vi "Current_Calib_Filenames.vi"(3 "Calib Filename":path[](array[path]), 4 "Channel ID input":string[](array[string]), 5 "Mode":T1) -> (0 "Calib Filename Out":path[](array[path]), 1 "Channel ID Output":string[](array[string]))   [LabVIEW 2017]
uses:
  Controls/App_Global.ctl
  File/Setup_Filetype.ctl
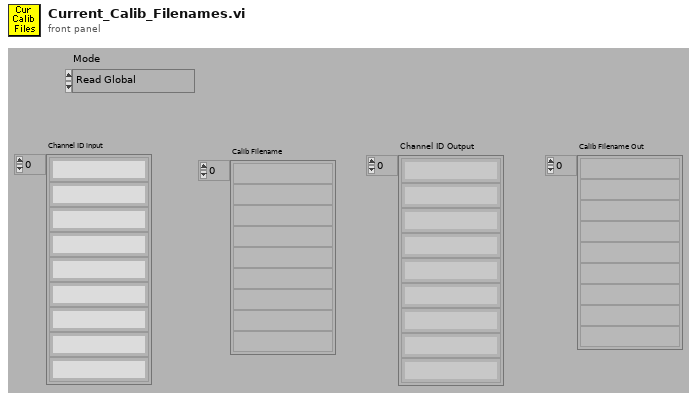
[diagram p1: front panel]
types:
  T1 = typedef "App_Global.ctl" = enum16{"Read Global", "Write to Global", "Initialise Array"}
  T2 = typedef "Setup_Filetype.ctl" = enum16{"Measurement Setups", "Calibration Setups", "General", "Results File Plotter Setups", "Speed Calib Tweaks"}
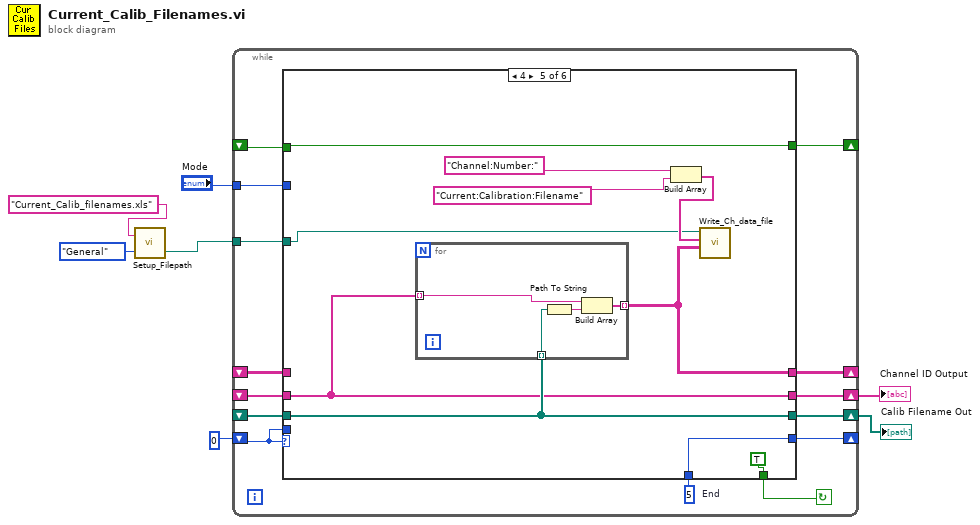
[diagram p0: block diagram]
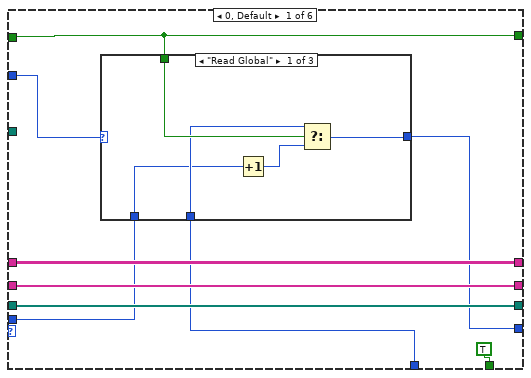
[diagram p2: hidden frame]
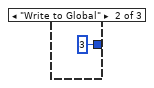
[diagram p3: hidden frame]
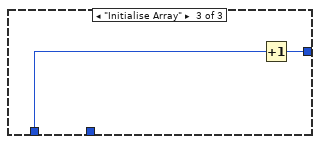
[diagram p4: hidden frame]
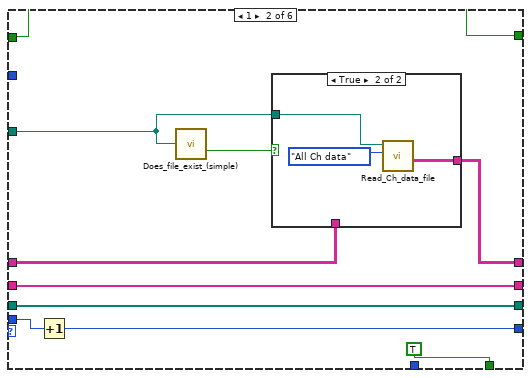
[diagram p5: hidden frame]
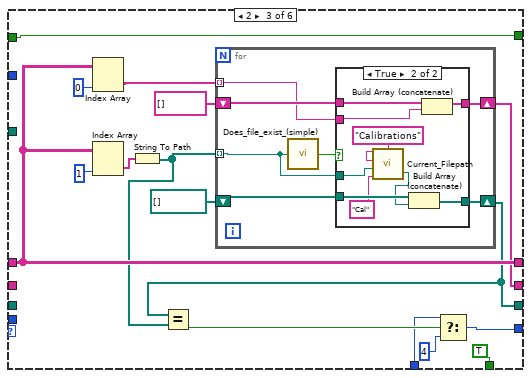
[diagram p7: hidden frame]
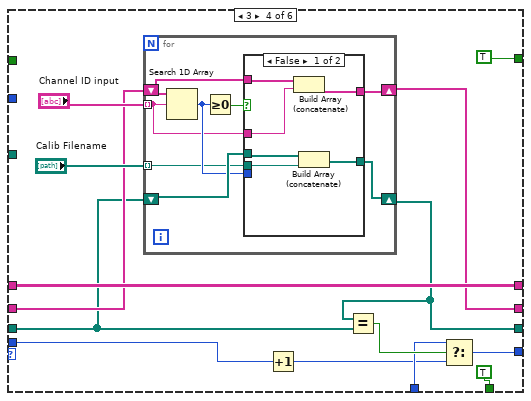
[diagram p9: hidden frame]
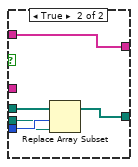
[diagram p10: hidden frame]
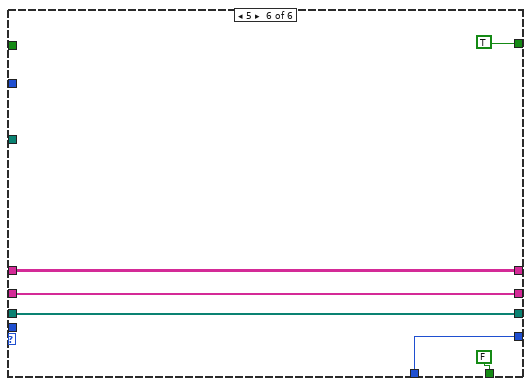
[diagram p11: hidden frame]
diagram:
  n1 = call "Setup_Filepath.vi"("Setup File Type"=Setup_Filetype."General", "Filename in"="Current_Calib_filenames.xls" ("Substring")) -> ("Filename Out"=w2:path)  [unwired: 1 out]
  n2 = while {
    shift-left: _ -> [w10]
    shift-right: [w12] -> w4
    shift-left: _ -> [w11]
    shift-right: [w13] -> w5
    tunnel: "Mode" -> [w17]
    shift-left: 0 -> [w18]
    shift-right: [w19] -> _
    shift-left: _ -> [w14]
    shift-right: [w15] -> _
    shift-left: _ -> [w21]
    shift-right: [w16] -> _
    tunnel: w2 -> [w8]
    stop <- w20 continue-if-true
    w9 = 5  # End
    n3 = case shown="4" w18 {
      tunnel: w21 -> [w25 w45 w64 _ w129 _]
      tunnel: [TRUE TRUE TRUE TRUE TRUE FALSE] -> w20
      tunnel: [w22 w46 w56 w87 w128 w135] -> w19
      tunnel: w18 -> [w23 w47 _ w89 _ _]
      tunnel: w17 -> [w26 _ _ _ _ _]
      tunnel: [w25 w45 w64 TRUE w129 TRUE] -> w16
      tunnel: [w28 w43 w63 w99 w121 w138] -> w15
      tunnel: w14 -> [w28 w42 w63 w99 _ w138]
      tunnel: [w30 w41 w61 w94 w122 w137] -> w13
      tunnel: [w29 w40 w60 w93 w123 w136] -> w12
      tunnel: w11 -> [w30 w41 _ w95 w122 w137]
      tunnel: w10 -> [w29 w40 _ w92 w123 w136]
      tunnel: w9 -> [w24 _ w57 w90 w128 w135]
      tunnel: w8 -> [_ w39 _ _ w120 _]
      frame 0, Default {
        n4 = case shown="\"Read Global\"" w26 {
          tunnel: w25 -> [w35 _ _]
          tunnel: w24 -> [w34 _ _]
          tunnel: w23 -> [w32 _ w38]
          tunnel: [w31 3 ("End") w37] -> w22
          frame "Read Global" {
            n5 = Increment(x=w32) -> (x+1=w33:i32)
            n6 = Select(t=w34, s=w35, f=w33) -> (s? t:f=w31:i32)
          }
          frame "Write to Global" {
          }
          frame "Initialise Array" {
            n7 = Increment(x=w38) -> (x+1=w37:i32)
          }
        }
      }
      frame 1 {
        n8 = Increment(x=w47) -> (x+1=w46:i32)
        n9 = call "Does_file_exist_(simple).vi"("Pathname"=w39) -> ("exists?"=w44:bool)
        n10 = case shown="True" w44 {
          tunnel: w39 -> [_ w51]
          tunnel: [w49 w50] -> w43
          tunnel: w42 -> [w49 _]
          frame False {
          }
          frame True {
            n11 = call "Read_Ch_data_file.vi"("Output"=enum16{"All Ch data", "The last few rows"}."All Ch data", "Filename"=w51) -> ("Channel Values"=w50:string[][])  [unwired: 3 in, 4 out]
          }
        }
      }
      frame 2 {
        n12 = Index Array(array=w63, index (col)=0 ("Index")) -> (element=w54:string[])  [unwired: 1 in]
        n13 = Index Array(array=w63, index (col)=1 ("Index")) -> (element=w65:string[])  [unwired: 1 in]
        n14 = String To Path(string=w65) -> (path=w59:path[])
        n15 = for {
          shift-right: [w73] -> w61
          shift-right: [w70] -> w60
          shift-left: path[] [] -> [w71]
          tunnel: w59 -> [w69] mode=indexing
          shift-left: string[] [] -> [w74]
          tunnel: w54 -> [w72] mode=indexing
          n16 = call "Does_file_exist_(simple).vi"("Pathname"=w69) -> ("exists?"=w75:bool)
          n17 = case shown="True" w75 {
            tunnel: w74 -> [w77 w86]
            tunnel: [w77 w85] -> w73
            tunnel: w72 -> [_ w78]
            tunnel: w71 -> [w76 w84]
            tunnel: [w76 w83] -> w70
            tunnel: w69 -> [_ w82]
            frame False {
            }
            frame True {
              n18 = call "Current_Filepath.vi"("Short_Name"="Cal", "Filename in"=w82, "Data Type"="Calibrations") -> ("Filename Out"=w80:path)  [unwired: 1 in, 1 out]
              n19 = Build Array (concatenate)(w84, w80) -> (w83:path[])
              n20 = Build Array (concatenate)(w86, w78) -> (w85:string[])
            }
          }
        }
        n21 = Equal?(x=w60, y=w59) -> (x = y?=w58:bool)
        n22 = Select(t=w57, s=w58, f=4) -> (s? t:f=w56:i32)
      }
      frame 3 {
        n23 = for {
          tunnel: "Channel ID input" -> [w101] mode=indexing
          shift-right: [w104] -> w93
          shift-left: w92 -> [w107]
          tunnel: "Calib Filename" -> [w105] mode=indexing
          shift-right: [w103] -> w94
          shift-left: w95 -> [w102]
          n24 = Search 1D Array(1D array=w102, element=w101) -> (index of element=w106:i32)  [unwired: 1 out]
          n25 = Greater Or Equal To 0?(x=w106) -> (x >= 0?=w108:bool)
          n26 = case shown="False" w108 {
            tunnel: w107 -> [w111 w119]
            tunnel: w106 -> [_ w118]
            tunnel: w105 -> [w110 w117]
            tunnel: [w109 w116] -> w104
            tunnel: [w112 w115] -> w103
            tunnel: w102 -> [w114 w115]
            tunnel: w101 -> [w113 _]
            frame False {
              n27 = Build Array (concatenate)(w114, w113) -> (w112:string[])
              n28 = Build Array (concatenate)(w111, w110) -> (w109:path[])
            }
            frame True {
              n29 = Replace Array Subset(array=w119, new element=w117, index=w118) -> (w116:path[])
            }
          }
        }
        n30 = Increment(x=w89) -> (x+1=w88:i32)
        n31 = Equal?(x=w93, y=w92) -> (x = y?=w91:bool)
        n32 = Select(t=w90, s=w91, f=w88) -> (s? t:f=w87:i32)
      }
      frame 4 {
        n33 = for {
          tunnel: w123 -> [w133] mode=indexing
          tunnel: w122 -> [w130] mode=indexing
          tunnel: [w132] -> w121 mode=indexing
          n34 = Path To String(path=w133) -> (string=w131:string)
          n35 = Build Array(w130, w131) -> (w132:string[])
        }
        n36 = Build Array("Channel:Number:", "Current:Calibration:Filename") -> (w124:string[])
        n37 = call "Write_Ch_data_file.vi"("Channel Values"=w121, "Channel names"=w124, "Filename"=w120) -> ()  [unwired: 5 in, 4 out]
      }
      frame 5 {
      }
    }
  }
  "Channel ID Output" <- w5
  "Calib Filename Out" <- w4
